vi "sub_gist11.vi"(1 "hist2":cluster{i16[], i32[]}, 2 "hist1":cluster{i16[], i32[]}) -> (0 "hist1-2":cluster{i16[], i32[]})   [LabVIEW 2010]
panel:
  # "Вычитание двух гистограмм"
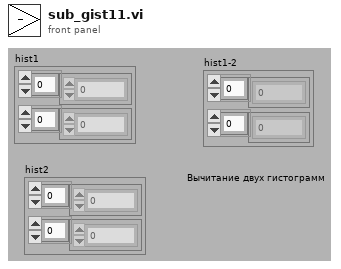
[diagram p1: front panel]
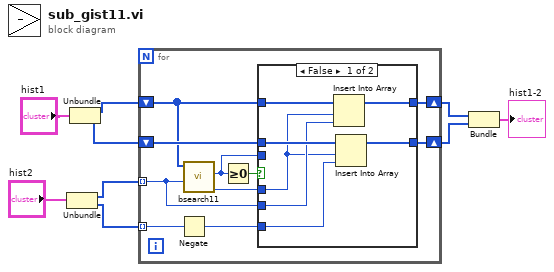
[diagram p0: block diagram]
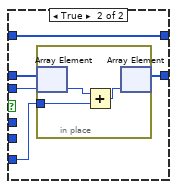
[diagram p2: hidden frame]
diagram:
  n1 = Unbundle("hist2") -> (w7:i16[], w6:i32[])
  n2 = Unbundle("hist1") -> (w5:i16[], w4:i32[])
  n3 = for {
    tunnel: w7 -> [w12] mode=indexing
    tunnel: w6 -> [w17] mode=indexing
    shift-right: [w14] -> w3
    shift-left: w5 -> [w13]
    shift-right: [w15] -> w2
    shift-left: w4 -> [w18]
    n4 = Negate(x=w17) -> (-x=w10:i32)
    n5 = call "bsearch11.vi"("val"=w12, "Array"=w13) -> ("a"=w11:i32, "idx"=w16:i32)  [unwired: 4 in]
    n6 = Greater Or Equal To 0?(x=w16) -> (x >= 0?=w19:bool)
    n7 = case shown="False" w19 {
      tunnel: w18 -> [w24 w31]
      tunnel: w10 -> [w21 w30]
      tunnel: w16 -> [_ w29]
      tunnel: [w23 w28] -> w15
      tunnel: [w25 w27] -> w14
      tunnel: w13 -> [w26 w27]
      tunnel: w12 -> [w22 _]
      tunnel: w11 -> [w20 _]
      frame False {
        n8 = Insert Into Array(array=w26, index=w20, new element=w22) -> (w25:i16[])
        n9 = Insert Into Array(array=w24, index=w20, new element=w21) -> (w23:i32[])
      }
      frame True {
        n10 = in-place {
          in-place-border: w30 -> [w32]
          n11 = in-place-array #1(w31, w29) -> (w34:i32)
          n12 = Add(x=w34, y=w32) -> (x+y=w33:i32)
          n13 = in-place-array #1(w33) -> (w28:i32[])  [unwired: 1 out]
        }
      }
    }
  }
  n14 = Bundle(w3, w2) -> (→"hist1-2":cluster{i16[], i32[]})  [unwired: 1 in]
